vi "inputGen.vi"(4 "Chemin du fichier":path=path "C:/Users/manip/Documents/Thermo aquisition data/labview/input/data.csv", 6 "Labview opt":T2={"Fréequence maximale (Hz)"=0.1, "Temps de simulation (min) 2"=2.0, "Amplitude minimale (V) 2"=0.0, "Amplitude maximale (V) 2"=1.0}, 7 "Fréequence \nd'échantillonage (alim)":dbl caption="Fréequence d'échantillonage (Hz)", 8 "Entrée d'erreur":errorcluster caption="Erreur IN", 9 "Commande onglets":enum32{"Labview", "CSV"}(tab), 11 "ID d'entrée":T1) -> (0 "Sortie d'erreur":errorcluster caption="Erreur OUT", 1 "Signal d'entrée":cluster{dbl[], dbl[]}(graph), 3 "ID de sortie":T1, 5 "DSP par FFT":cluster{dbl[], dbl[]}(graph))   [LabVIEW 2019]
uses:
  <vilib>/Utility/file.llb/Read Delimited Spreadsheet (DBL).vi
  <vilib>/Analysis/NI_AALPro.lvlib
panel:
  out "MaxFreqAff":dbl
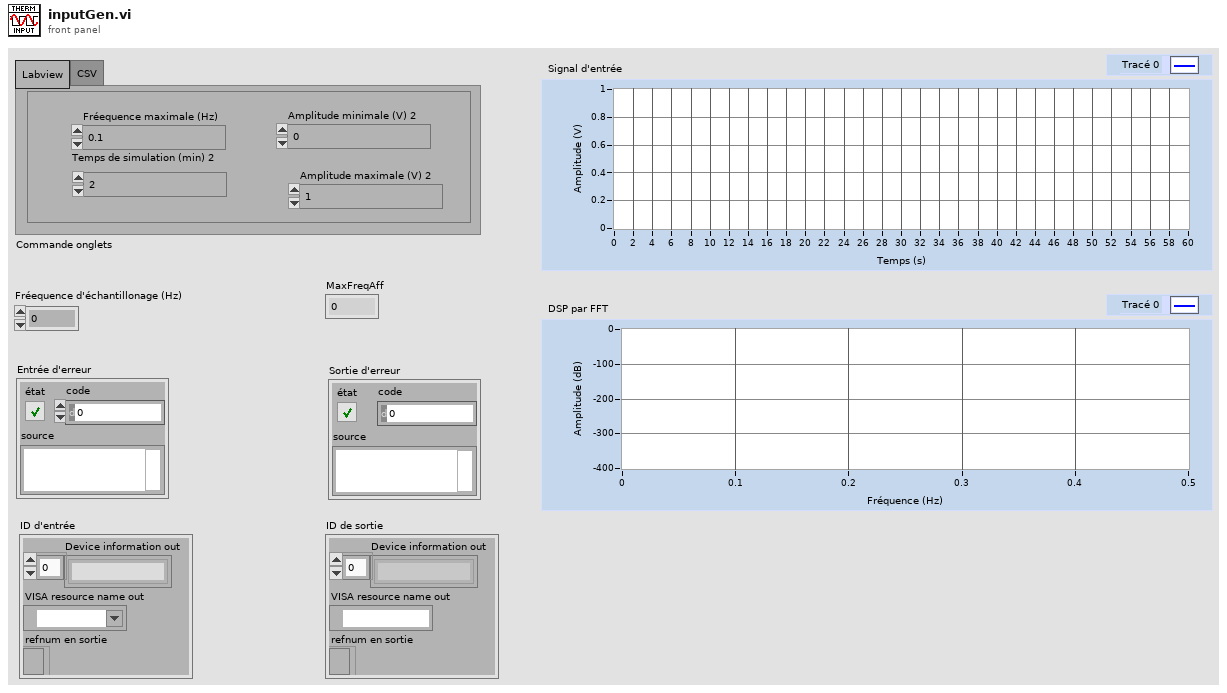
[diagram p1: front panel]
types:
  T1 = cluster{"Device information out":string[], "VISA resource name out":refnum<visa-resource-name>, "refnum en sortie":refnum<file>}
  T2 = cluster{"Fréequence maximale (Hz)":dbl, "Temps de simulation (min) 2":dbl, "Amplitude minimale (V) 2":dbl, "Amplitude maximale (V) 2":dbl}
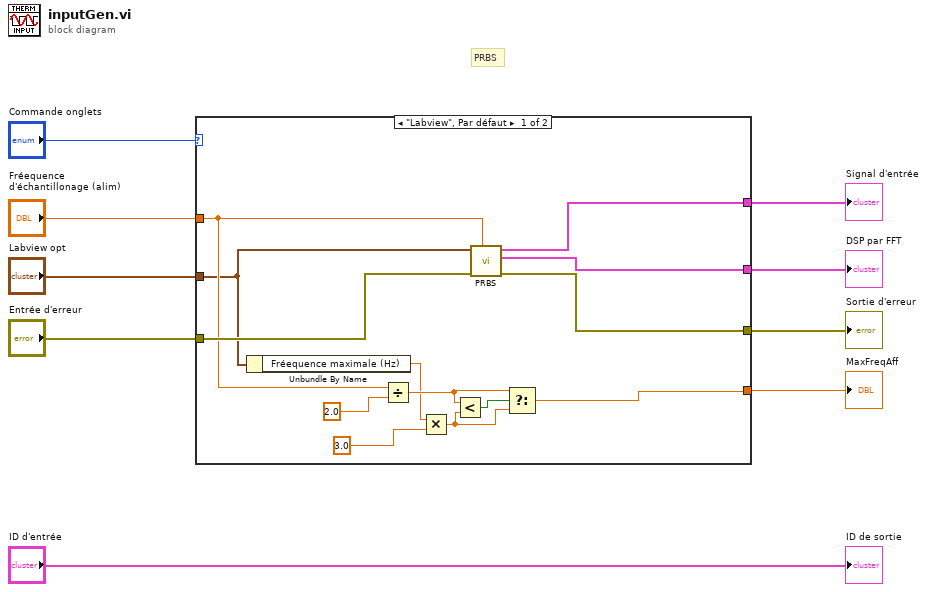
[diagram p0: block diagram]
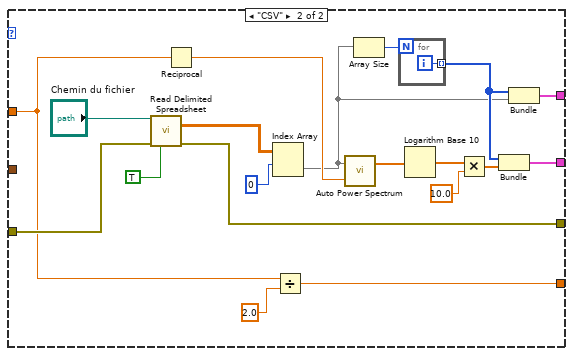
[diagram p2: hidden frame]
diagram:
  # "PRBS"
  n1 = case shown="\"Labview\", Par défaut" "Commande onglets" {
    tunnel: "Entrée d'erreur" -> [w22 w40]
    tunnel: "Fréequence \nd'échantillonage (alim)" -> [w16 w27]
    tunnel: "Labview opt" -> [w15 _]
    tunnel: [w13 w23] -> w2
    tunnel: [w12 w25] -> w3
    tunnel: [w11 w24] -> w5
    tunnel: [w10 w26] -> w4
    frame "Labview", Default {
      n2 = Unbundle By Name(w15) -> ("Fréequence maximale (Hz)"=w14:dbl)
      n3 = Divide(x=w16, y=2.0) -> (x/y=w21:dbl)
      n4 = Multiply(x=w14, y=3.0) -> (x*y=w19:dbl)
      n5 = Less?(x=w21, y=w19) -> (x < y?=w20:bool)
      n6 = call "PRBS.vi"("Fréquence \nd'echantillonage (Hz)"=w16, "Entrée d'erreur\n(sans erreur)"=w22, "Labview opt"=w15) -> ("Sorti d'erreur"=w12:errorcluster, "DSP par FFT"=w11:cluster{dbl[], dbl[]}, "u"=w10:cluster{dbl[], dbl[]})  [unwired: 6 in]
      n7 = Select(t=w21, s=w20, f=w19) -> (s? t:f=w13:dbl)
    }
    frame "CSV" {
      n8 = call-poly <vilib>:"Read Delimited Spreadsheet.vi"("file path (dialog if empty)"="Chemin du fichier", "error in (no error)"=w40, "transpose? (F)"=TRUE) -> ("all rows"=w31:dbl[][], "error out"=w25:errorcluster)  [unwired: 7 in, 4 out]
      n9 = Reciprocal(x=w27) -> (1/x=w35:dbl)
      n10 = Index Array(array=w31, index (row)=0 ("taille de la dimension")) -> (element=w29:dbl[])  [unwired: 1 in]
      n11 = Divide(x=w27, y=2.0) -> (x/y=w23:dbl)
      n12 = call <vilib>:"Auto Power Spectrum.vi"("dt"=w35, "Signal (V)"=w29) -> ("Power Spectrum (V^2 rms)"=w39:dbl[])  [unwired: 1 out]
      n13 = Array Size(array=w29) -> (size(s)=w34:i32)
      n14 = for {
        N: w34 -> [_]
        tunnel: [w42] -> w33 mode=indexing
        i -> [w42]
      }
      n15 = Logarithm Base 10(1:w39) -> (0:w36:dbl[])
      n16 = Multiply(x=w36, y=10.0 ("x")) -> (x*y=w37:dbl[])
      n17 = Bundle(w33, w37) -> (w24:cluster{i32[], dbl[]})  [unwired: 1 in]
      n18 = Bundle(w33, "all rows"=w29) -> (w26:cluster{i32[], "all rows":dbl[]})  [unwired: 1 in]
    }
  }
  "Sortie d'erreur" <- w3
  "DSP par FFT" <- w5
  "Signal d'entrée" <- w4
  "MaxFreqAff" <- w2
  "ID de sortie" <- "ID d'entrée"
